vi "步进电机控制.vi"() -> ()   [LabVIEW 2015]
doc: "本范例使用Labview作为F4-Pro上位机控制步进电机.,可以使用速度模式,点动模式控制步进电机,同时检测限位开关的状态,可以配置通用输出端口的电平."
uses:
  <vilib>/Platform/browser.llb/Open URL in Default Browser (string).vi
  lib/pcomm/PCOMM.lvlib
panel:
  out "字符串 5":string="位置速度"
  out "字符串 4":string="运动控制"
  out "字符串 3":string="通用输入输出"
  out "字符串 2":string="运动模式"
  in  "刷新按钮":bool
  out "字符串":string="串口设置"
  in  "速度调节":sgl(knob) caption="速度旋钮" min=-600 max=600 scale=-600.0..600.0 scale format="%#_3f"
  in  "打开/关闭串口":bool
  in  "串口号":i32(ring)=1 items=["COM1 通信端口 (COM1)"=1, "COM2 ELTIMA Virtual Serial Port (COM2->COM3)"=2, "COM3 ELTIMA Virtual Serial Port (COM3->COM2)"=3, "COM8 USB-SERIAL CH340 (COM8)"=8]
  in  "波特率":i32(ring)=16 items=["1800"=8, "2400"=9, "4800"=10, "7200"=11, "9600"=12, "19200"=13, "38400"=14, "57600"=15, "115200"=16, "230400"=17, "460800"=18, "921600"=19]
  in  "数据比特":i32(ring)=3 caption="数据位" items=["5", "6", "7", "8"]
  in  "停止位":i32(ring) items=["1"=0, "2"=4]
  in  "奇偶校验":i32(ring) caption="校   验" items=["None"=0, "Odd"=8, "Even"=24, "Mark"=40, "Space"=56]
  in  "发送位置":bool
  in  "细分数":u32(ring)=32 items=["1"=1, "2"=2, "4"=4, "8"=8, "16"=16, "32"=32, "64"=64, "128"=128]
  out "圈数":sgl
  in  "脉冲数":u32 step=1
  in  "Out4":T1
  in  "Out3":T1
  in  "Out2":T1
  in  "Out1":T1
  out "IN3":bool caption="正极限"
  out "IN1":bool caption="原点检测"
  out "IN2":bool caption="负极限"
  in  "响应测试":bool
  in  "停止按钮":bool
  in  "点动控制":bool
  in  "接收:":string="硬石电子http://www.ing10bbs.com/\n            携手合作,共创未来\n"
  in  "速度位置选择":enum32{"未选择", "速度模式", "位置模式"}(radio)
  # "概述：Labview控制步进电机例程\n要求：PC已安装串口驱动，F4-Pro已下载配套例程.\n操作步骤：\n1.  使用USB线连接到F4-Pro的调试串口接口。\n2.  确保串口号为连接到F4-Pro的串口。\n3.  配置波特率等信息，F4-Pro通信配置是115200-8-None-1。\n4.  打开串口。\n5.  点击响应测试测试连接，文本框提示连接成功。"
  # "6.  选择速度模式或者位置模式\n7.  如果选择速度模式,则拖动速度旋钮，设置速度，\n    也可以直接输入速度值。\n8.  如果选择位置模式,则设置脉冲数和细分数，点击发送位置按钮。\n9.  按下点动控制按钮，则电机转动，松开按钮则停止，\n     速度值为旋钮所设置的速度值。\n10. 点击Out1~4，可以控制通用输出端口电平\n11. IN1~3指示通用输入1~3的电平状态"
  # "RPM"
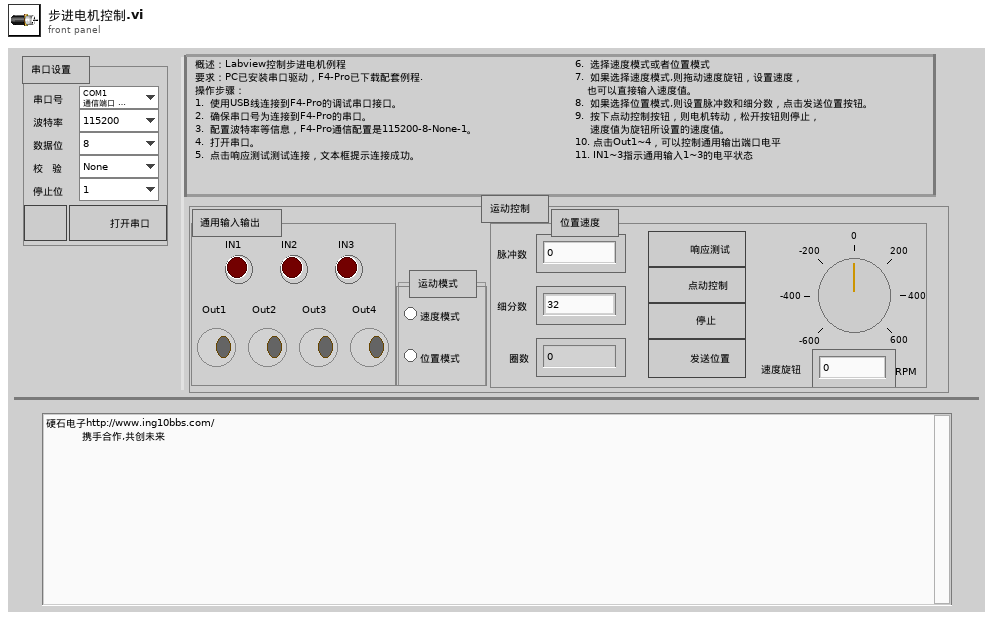
[diagram p1: front panel]
types:
  T1 = typedef "控件_通用输出.ctl" = bool
  T2 = enum8{"Enabled", "Disabled", "Disabled and Grayed Out"}
  T3 = typedef "控件 1" = bool
  T4 = typedef "LVRectTypeDef.ctl" = cluster{"Left":i16, "Top":i16, "Right":i16, "Bottom":i16}
  T5 = typedef "LVPointTypeDef.ctl" = cluster{"Horizontal":i16, "Vertical":i16}
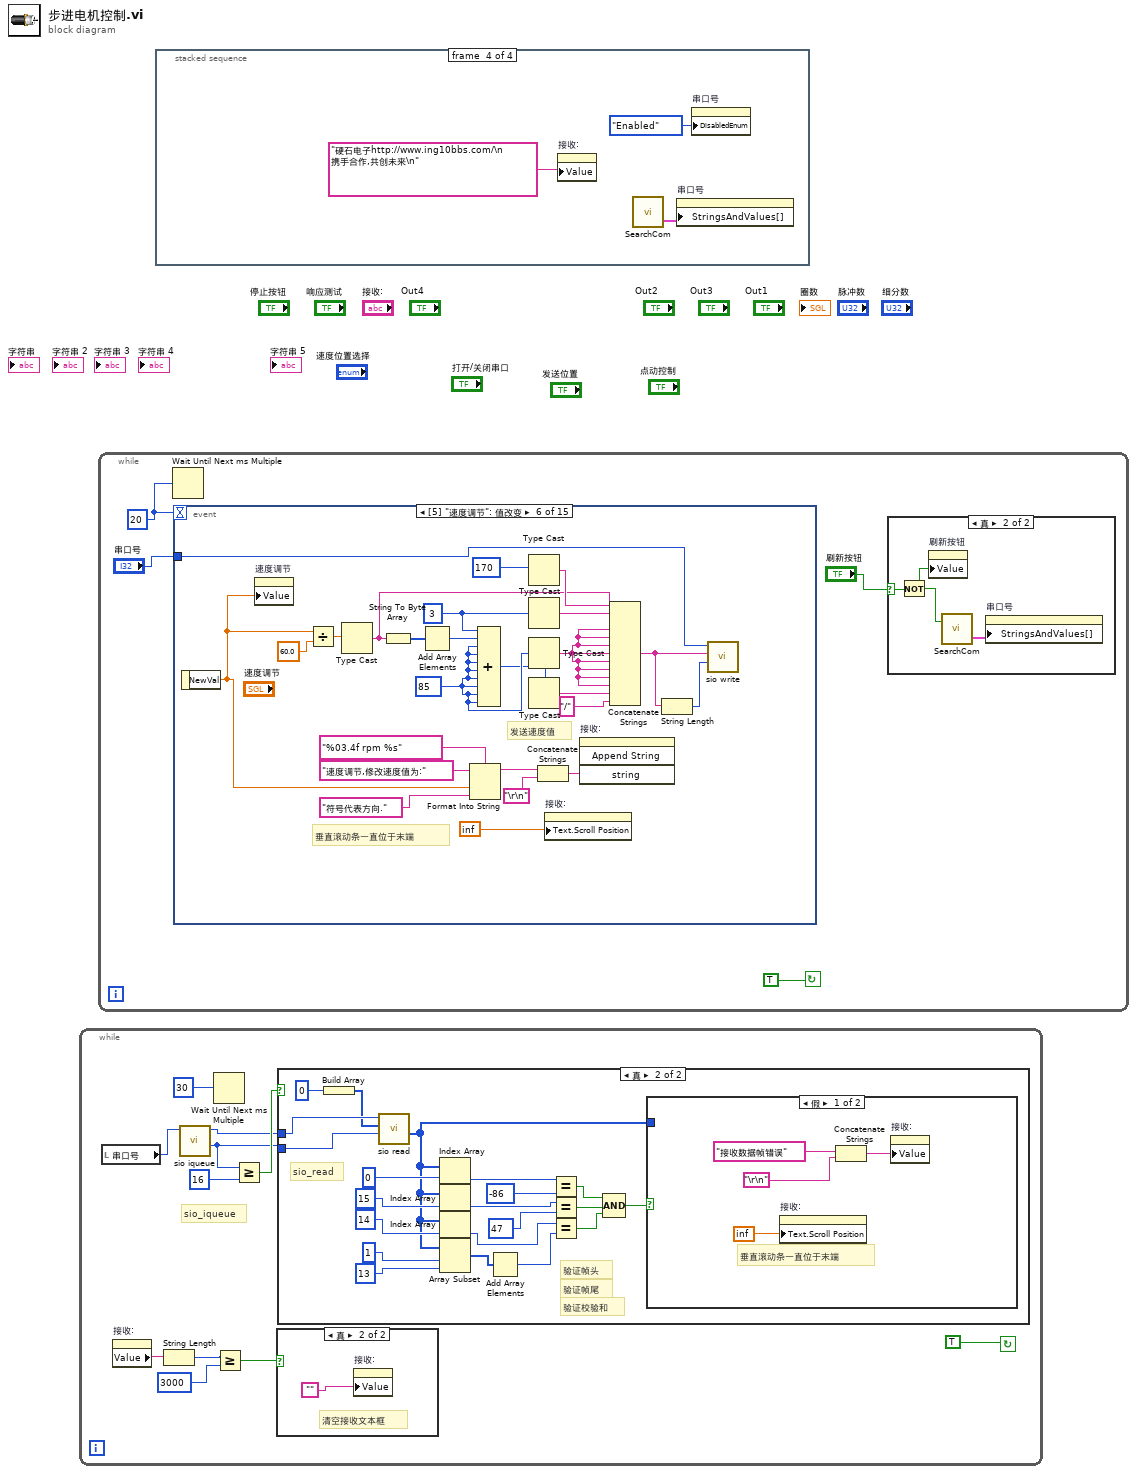
[diagram p0: block diagram]
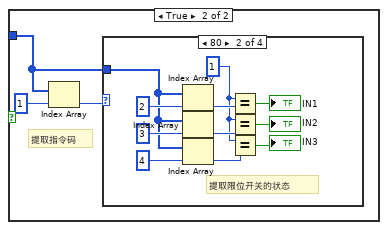
[diagram p4: hidden frame]
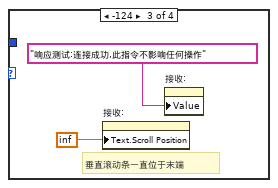
[diagram p6: hidden frame]
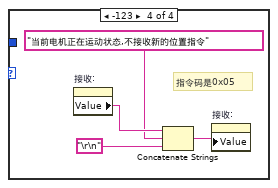
[diagram p7: hidden frame]
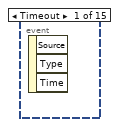
[diagram p9: hidden frame]
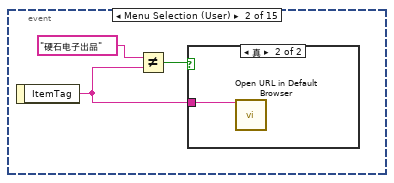
[diagram p10: hidden frame]
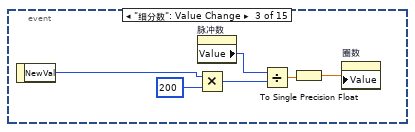
[diagram p12: hidden frame]
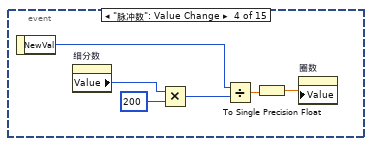
[diagram p13: hidden frame]
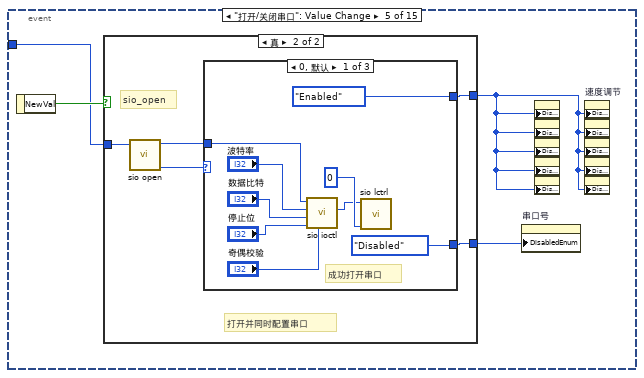
[diagram p14: hidden frame]
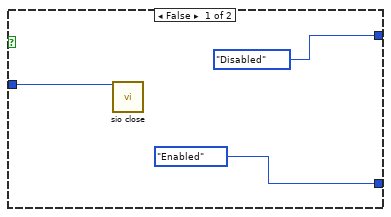
[diagram p15: hidden frame]
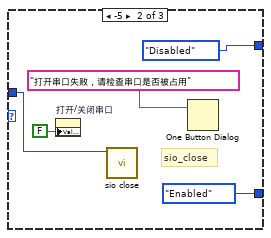
[diagram p16: hidden frame]
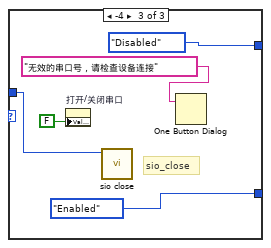
[diagram p17: hidden frame]
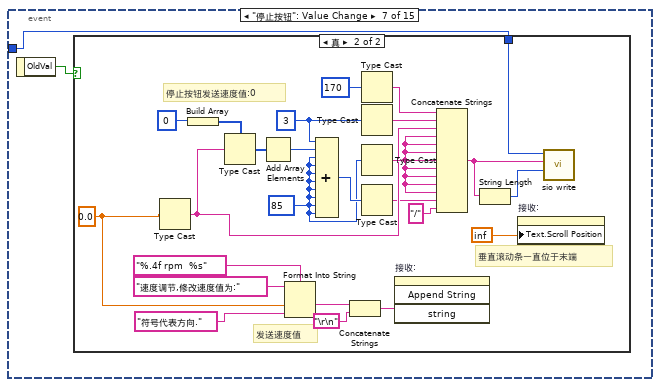
[diagram p18: hidden frame]
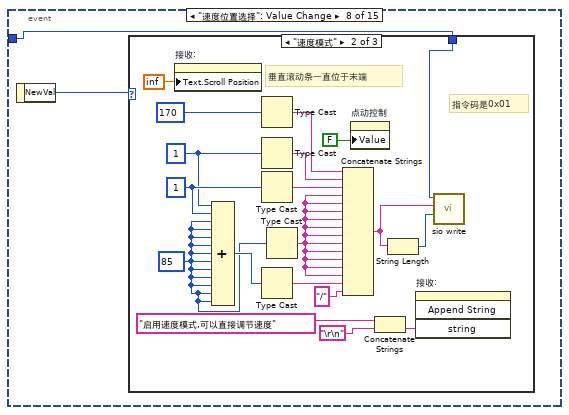
[diagram p20: hidden frame]
diagram:
  n1 = while {
    stop <- TRUE continue-if-true
    # "sio_iqueue"
    n2 = local read "串口号"() -> (w2:i32)
    n3 = property on="接收:" class="Str"() -> ("Value"=w3:string)  [unwired: 2 in, 2 out]
    n4 = String Length(string=w3) -> (length=w4:i32)
    n5 = call "sio iqueue.vi"("port"=w2) -> ("len"=w7:i32, "port"=w1:i32)  [unwired: 8 in, 1 out]
    n6 = Wait Until Next ms Multiple(millisecond multiple=u32 30) -> ()  [unwired: 1 out]
    n7 = Greater Or Equal?(x=w4, y=3000) -> (x >= y?=w5:bool)
    n8 = Greater Or Equal?(x=w7, y=16) -> (x >= y?=w8:bool)
    n9 = case shown="真" w5 {
      frame False {
      }
      frame True {
        # "清空接收文本框"
        n10 = property on="接收:" class="Str"("Value"="") -> ()  [unwired: 2 in, 2 out]
      }
    }
    n11 = case shown="真" w8 {
      tunnel: w1 -> [_ w15]
      tunnel: w7 -> [_ w13]
      frame False {
      }
      frame True {
        # "sio_read"
        # "验证帧尾"
        # "验证校验和"
        # "验证帧头"
        n12 = Build Array(i8 0) -> (w14:i8[])
        n13 = call "sio read.vi"("len"=w13, "buf"=w14, "port"=w15) -> ("buf out"=w16:i8[])  [unwired: 4 in, 3 out]
        n14 = Index Array(array=w16, index=0) -> (element=w31:i8)
        n15 = Index Array(array=w16, index=15) -> (element=w18:i8)
        n16 = Index Array(array=w16, index=14) -> (element=w20:i8)
        n17 = Array Subset(array=w16, index=1, length=13) -> (w24:i8[])
        n18 = Add Array Elements(numeric array=w24) -> (sum=w19:i8)
        n19 = Equal?(x=w31, y=i8 -86) -> (x = y?=w29:bool)
        n20 = Equal?(x=w18, y=i8 47) -> (x = y?=w26:bool)
        n21 = Equal?(x=w20, y=w19) -> (x = y?=w22:bool)
        n22 = Compound Arithmetic op=AND ("复合运算")(w29, w26, w22) -> (w33:bool)
        n23 = case shown="假" w33 {
          tunnel: w16 -> [_ w38]
          frame False {
            # "垂直滚动条一直位于末端"
            n24 = property on="接收:" class="Str"("Text.Scroll Position"=inf) -> ()  [unwired: 2 in, 2 out]
            n25 = Concatenate Strings("接收数据帧错误", "\r\n") -> (w35:string)
            n26 = property on="接收:" class="Str"("Value"=w35) -> ()  [unwired: 2 in, 2 out]
          }
          frame True {
            # "提取指令码"
            n27 = Index Array(array=w38, index=1) -> (element=w39:i8)
            n28 = case shown="80" w39 {
              tunnel: w38 -> [_ w44 _ _]
              frame Default {
                # "指令码0x00,无效"
              }
              frame -128 {
                w41 = i8 1
                # "提取限位开关的状态"
                n29 = Index Array(array=w44, index=2) -> (element=w47:i8)
                n30 = Index Array(array=w44, index=3) -> (element=w43:i8)
                n31 = Index Array(array=w44, index=4) -> (element=w42:i8)
                n32 = Equal?(x=w41, y=w47) -> (x = y?=→"IN1":bool)
                n33 = Equal?(x=w41, y=w43) -> (x = y?=→"IN2":bool)
                n34 = Equal?(x=w41, y=w42) -> (x = y?=→"IN3":bool)
              }
              frame -124 {
                # "垂直滚动条一直位于末端"
                n35 = property on="接收:" class="Str"("Text.Scroll Position"=inf) -> ()  [unwired: 2 in, 2 out]
                n36 = property on="接收:" class="Str"("Value"="响应测试:连接成功,此指令不影响任何操作") -> ()  [unwired: 2 in, 2 out]
              }
              frame -123 {
                # "指令码是0x05"
                n37 = property on="接收:" class="Str"() -> ("Value"=w57:string)  [unwired: 2 in, 2 out]
                n38 = Concatenate Strings(w57, "当前电机正在运动状态,不接收新的位置指令", "\r\n") -> (w56:string)
                n39 = property on="接收:" class="Str"("Value"=w56) -> ()  [unwired: 2 in, 2 out]
              }
            }
          }
        }
      }
    }
  }
  n40 = while {
    stop <- TRUE continue-if-true
    w60 = 20
    n41 = Wait Until Next ms Multiple(millisecond multiple=w60) -> ()  [unwired: 1 out]
    n42 = event shown="[5] \"速度调节\": 值改变" {
      selector: _ -> [_ _ _ _ _ _ _ _ _ _ _ _ _ _ _]
      dyn-events: _ -> [_ _ _ _ _ _ _ _ _ _ _ _ _ _ _]
      timeout: w60 -> [_ _ _ _ _ _ _ _ _ _ _ _ _ _ _]
      tunnel: "串口号" -> [_ _ _ _ w82 w114 w137 w164 w221 w261 w277 w305 w333 w361 w388]
      event Timeout {
        n43 = event-data() -> ()  [unwired: 1 in, 3 out]
      }
      event Menu Selection (User) {
        n44 = event-data() -> ("ItemTag"=w65:string)  [unwired: 1 in]
        n45 = Not Equal?(x="硬石电子出品", y=w65) -> (x != y?=w66:bool)
        n46 = case shown="真" w66 {
          tunnel: w65 -> [_ w68]
          frame False {
          }
          frame True {
            n47 = call-poly <vilib>:"Open URL in Default Browser.vi"("URL"=w68) -> ()  [unwired: 5 in, 2 out]
          }
        }
      }
      event "细分数": Value Change {
        n48 = event-data() -> ("NewVal"=w69:u32)  [unwired: 1 in]
        n49 = Multiply(x=w69, y=200) -> (x*y=w72:u32)
        n50 = property on="脉冲数" class="DigNum (严格)"() -> ("Value"=w74:u32)  [unwired: 2 in, 2 out]
        n51 = Divide(x=w74, y=w72) -> (x/y=w71:dbl)
        n52 = To Single Precision Float(number=w71) -> (single precision float=w70:sgl)
        n53 = property on="圈数" class="DigNum (严格)"("Value"=w70) -> ()  [unwired: 2 in, 2 out]
      }
      event "脉冲数": Value Change {
        n54 = event-data() -> ("NewVal"=w75:u32)  [unwired: 1 in]
        n55 = property on="细分数" class="Ring (严格)"() -> ("Value"=w80:u32)  [unwired: 2 in, 2 out]
        n56 = Multiply(x=w80, y=200) -> (x*y=w78:u32)
        n57 = Divide(x=w75, y=w78) -> (x/y=w77:dbl)
        n58 = To Single Precision Float(number=w77) -> (single precision float=w76:sgl)
        n59 = property on="圈数" class="DigNum (严格)"("Value"=w76) -> ()  [unwired: 2 in, 2 out]
      }
      event "打开/关闭串口": Value Change {
        n60 = event-data() -> ("NewVal"=w84:bool)  [unwired: 1 in]
        n61 = case shown="真" w84 {
          tunnel: [T2."Enabled" w92] -> w83
          tunnel: [T2."Disabled" w91] -> w81
          tunnel: w82 -> [w85 w90]
          frame False {
            n62 = call "sio close.vi"("port"=w85) -> ()  [unwired: 9 in, 2 out]
          }
          frame True {
            # "sio_open"
            # "打开并同时配置串口"
            n63 = call "sio open.vi"("port"=w90) -> ("port"=w88:i32, "Status"=w89:i32)  [unwired: 6 in]
            n64 = case shown="0, 默认" w89 {
              tunnel: w88 -> [w97 w102 w107]
              tunnel: [T2."Enabled" T2."Disabled" T2."Disabled"] -> w91
              tunnel: [T2."Disabled" T2."Enabled" T2."Enabled"] -> w92
              frame 0, Default {
                # "成功打开串口"
                n65 = call "sio ioctl.vi"("parity"="奇偶校验", "stop bits"="停止位", "data bits"="数据比特", "baud"="波特率", "port"=w97) -> ("port"=w93:i32)  [unwired: 5 in, 1 out]
                n66 = call "sio lctrl.vi"("mode"=0, "port"=w93) -> ()  [unwired: 8 in, 2 out]
              }
              frame -5 {
                # "sio_close"
                n67 = property on="打开/关闭串口" class="Bool (严格)"("Value"=FALSE) -> ()  [unwired: 2 in, 2 out]
                n68 = call "sio close.vi"("port"=w102) -> ()  [unwired: 9 in, 2 out]
                n69 = One Button Dialog(message="打开串口失败，请检查串口是否被占用") -> ()  [unwired: 1 in, 1 out]
              }
              frame -4 {
                # "sio_close"
                n70 = property on="打开/关闭串口" class="Bool (严格)"("Value"=FALSE) -> ()  [unwired: 2 in, 2 out]
                n71 = call "sio close.vi"("port"=w107) -> ()  [unwired: 9 in, 2 out]
                n72 = One Button Dialog(message="无效的串口号，请检查设备连接") -> ()  [unwired: 1 in, 1 out]
              }
            }
          }
        }
        n73 = property on="串口号" class="Ring (严格)"("DisabledEnum"=w83) -> ()  [unwired: 2 in, 2 out]
        n74 = property on="点动控制" class="Bool (严格)"("DisabledEnum"=w81) -> ()  [unwired: 2 in, 2 out]
        n75 = property on="Output2" class="Bool (严格)"("DisabledEnum"=w81) -> ()  [unwired: 2 in, 2 out]
        n76 = property on="速度位置选择" class="RadioBtnsControl (严格)"("DisabledEnum"=w81) -> ()  [unwired: 2 in, 2 out]
        n77 = property on="停止按钮" class="Bool (严格)"("DisabledEnum"=w81) -> ()  [unwired: 2 in, 2 out]
        n78 = property on="Output4" class="Bool (严格)"("DisabledEnum"=w81) -> ()  [unwired: 2 in, 2 out]
        n79 = property on="速度调节" class="Knob (严格)"("DisabledEnum"=w81) -> ()  [unwired: 2 in, 2 out]
        n80 = property on="Output3" class="Bool (严格)"("DisabledEnum"=w81) -> ()  [unwired: 2 in, 2 out]
        n81 = property on="发送位置" class="Bool (严格)"("DisabledEnum"=w81) -> ()  [unwired: 2 in, 2 out]
        n82 = property on="响应测试" class="Bool (严格)"("DisabledEnum"=w81) -> ()  [unwired: 2 in, 2 out]
        n83 = property on="Output1" class="Bool (严格)"("DisabledEnum"=w81) -> ()  [unwired: 2 in, 2 out]
      }
      event "速度调节": Value Change {
        w124 = u8 85
        w123 = u8 3
        # "垂直滚动条一直位于末端"
        # "发送速度值"
        n84 = event-data() -> ("NewVal"=w117:sgl)  [unwired: 1 in]
        n85 = property on="速度调节" class="Knob (严格)"("Value"=w117) -> ()  [unwired: 2 in, 2 out]
        n86 = Divide(x=w117, y=sgl 60.0) -> (x/y=w136:sgl)
        n87 = Type Cast(x=w136) -> (*(type *) &x=w113:string)  [unwired: 1 in]
        n88 = String To Byte Array(string=w113) -> (unsigned byte array=w112:u8[])
        n89 = Add Array Elements(numeric array=w112) -> (sum=w128:u8)
        n90 = Format Into String(format string="%03.4f rpm %s", initial string="速度调节,修改速度值为:", w117, "符号代表方向.") -> (resulting string=w132:string)  [unwired: 1 in, 1 out]
        n91 = Compound Arithmetic op=ADD(w123, w128, w124, w124, w124, w124, w124, w124, w124, w124) -> (w120:u8)
        n92 = Type Cast(x=u8 170) -> (*(type *) &x=w121:string)  [unwired: 1 in]
        n93 = Type Cast(x=w123) -> (*(type *) &x=w122:string)  [unwired: 1 in]
        n94 = Type Cast(x=w124) -> (*(type *) &x=w126:string)  [unwired: 1 in]
        n95 = Type Cast(x=w120) -> (*(type *) &x=w127:string)  [unwired: 1 in]
        n96 = Concatenate Strings(w132, "\r\n") -> (w118:string)
        n97 = property on="接收:" class="Str"("Text.Scroll Position"=inf) -> ()  [unwired: 2 in, 2 out]
        n98 = invoke on="接收:" class="Str" method="Append String"("string"=w118) -> ()  [unwired: 3 in, 4 out]
        n99 = Concatenate Strings(w121, w122, w113, w126, w126, w126, w126, w126, w126, w126, w126, w127, "/") -> (w116:string)
        n100 = String Length(string=w116) -> (length=w115:i32)
        n101 = call "sio write.vi"("len"=w115, "buf"=w116, "port"=w114) -> ()  [unwired: 6 in, 3 out]
      }
      event "停止按钮": Value Change {
        n102 = event-data() -> ("OldVal"=w138:bool)  [unwired: 1 in]
        n103 = case shown="真" w138 {
          tunnel: w137 -> [_ w141]
          frame False {
          }
          frame True {
            w158 = u8 85
            w159 = u8 3
            w142 = sgl 0.0
            # "垂直滚动条一直位于末端"
            # "发送速度值"
            # "停止按钮发送速度值:0"
            n104 = Type Cast(x=w142) -> (*(type *) &x=w151:string)  [unwired: 1 in]
            n105 = Build Array(u8 0) -> (w154:u8[])
            n106 = Type Cast(type=w154, x=w151) -> (*(type *) &x=w153:u8[])
            n107 = Add Array Elements(numeric array=w153) -> (sum=w152:u8)
            n108 = Format Into String(format string="%.4f rpm  %s", initial string="速度调节,修改速度值为:", w142, "符号代表方向.") -> (resulting string=w145:string)  [unwired: 1 in, 1 out]
            n109 = Compound Arithmetic op=ADD(w159, w152, w158, w158, w158, w158, w158, w158, w158, w158) -> (w162:u8)
            n110 = Concatenate Strings(w145, "\r\n") -> (w143:string)
            n111 = Type Cast(x=u8 170) -> (*(type *) &x=w161:string)  [unwired: 1 in]
            n112 = Type Cast(x=w159) -> (*(type *) &x=w160:string)  [unwired: 1 in]
            n113 = Type Cast(x=w158) -> (*(type *) &x=w156:string)  [unwired: 1 in]
            n114 = Type Cast(x=w162) -> (*(type *) &x=w150:string)  [unwired: 1 in]
            n115 = invoke on="接收:" class="Str" method="Append String"("string"=w143) -> ()  [unwired: 3 in, 4 out]
            n116 = Concatenate Strings(w161, w160, w151, w156, w156, w156, w156, w156, w156, w156, w156, w150, "/") -> (w140:string)
            n117 = String Length(string=w140) -> (length=w139:i32)
            n118 = property on="接收:" class="Str"("Text.Scroll Position"=inf) -> ()  [unwired: 2 in, 2 out]
            n119 = call "sio write.vi"("len"=w139, "buf"=w140, "port"=w141) -> ()  [unwired: 6 in, 3 out]
          }
        }
      }
      event "速度位置选择": Value Change {
        n120 = event-data() -> ("NewVal"=w165:enum32{"未选择", "速度模式", "位置模式"})  [unwired: 1 in]
        n121 = case shown="\"速度模式\"" w165 {
          tunnel: w164 -> [w168 w186 w205]
          frame "未选择", Default {
            w169 = u8 85
            w174 = u8 0
            w175 = u8 1
            # "垂直滚动条一直位于末端"
            # "速度模式,指令码0x01"
            n122 = Compound Arithmetic op=ADD(w175, w174, w169, w169, w169, w169, w169, w169, w169, w169, w169, w169, w169) -> (w181:u8)
            n123 = Concatenate Strings("停止速度位置模式", "\r\n") -> (w170:string)
            n124 = Type Cast(x=u8 170) -> (*(type *) &x=w180:string)  [unwired: 1 in]
            n125 = Type Cast(x=w175) -> (*(type *) &x=w179:string)  [unwired: 1 in]
            n126 = Type Cast(x=w174) -> (*(type *) &x=w178:string)  [unwired: 1 in]
            n127 = Type Cast(x=w169) -> (*(type *) &x=w183:string)  [unwired: 1 in]
            n128 = Type Cast(x=w181) -> (*(type *) &x=w177:string)  [unwired: 1 in]
            n129 = invoke on="接收:" class="Str" method="Append String"("string"=w170) -> ()  [unwired: 3 in, 4 out]
            n130 = Concatenate Strings(w180, w179, w178, w183, w183, w183, w183, w183, w183, w183, w183, w183, w183, w183, w177, "/") -> (w167:string)
            n131 = String Length(string=w167) -> (length=w166:i32)
            n132 = property on="接收:" class="Str"("Text.Scroll Position"=inf) -> ()  [unwired: 2 in, 2 out]
            n133 = call "sio write.vi"("len"=w166, "buf"=w167, "port"=w168) -> ()  [unwired: 6 in, 3 out]
          }
          frame "速度模式" {
            w191 = u8 85
            w199 = u8 1
            w193 = u8 1
            # "垂直滚动条一直位于末端"
            # "指令码是0x01"
            n134 = property on="接收:" class="Str"("Text.Scroll Position"=inf) -> ()  [unwired: 2 in, 2 out]
            n135 = Compound Arithmetic op=ADD(w193, w199, w191, w191, w191, w191, w191, w191, w191, w191, w191, w191, w191) -> (w200:u8)
            n136 = Type Cast(x=u8 170) -> (*(type *) &x=w202:string)  [unwired: 1 in]
            n137 = Type Cast(x=w193) -> (*(type *) &x=w201:string)  [unwired: 1 in]
            n138 = Type Cast(x=w199) -> (*(type *) &x=w198:string)  [unwired: 1 in]
            n139 = Type Cast(x=w200) -> (*(type *) &x=w196:string)  [unwired: 1 in]
            n140 = Type Cast(x=w191) -> (*(type *) &x=w197:string)  [unwired: 1 in]
            n141 = Concatenate Strings(w202, w201, w198, w197, w197, w197, w197, w197, w197, w197, w197, w197, w197, w197, w196, "/") -> (w185:string)
            n142 = property on="点动控制" class="Bool (严格)"("Value"=FALSE) -> ()  [unwired: 2 in, 2 out]
            n143 = Concatenate Strings("启用速度模式,可以直接调节速度", "\r\n") -> (w187:string)
            n144 = String Length(string=w185) -> (length=w184:i32)
            n145 = invoke on="接收:" class="Str" method="Append String"("string"=w187) -> ()  [unwired: 3 in, 4 out]
            n146 = call "sio write.vi"("len"=w184, "buf"=w185, "port"=w186) -> ()  [unwired: 6 in, 3 out]
          }
          frame "位置模式" {
            w207 = u8 85
            w217 = u8 2
            w211 = u8 1
            # "垂直滚动条一直位于末端"
            # "指令码是0x01"
            n147 = property on="接收:" class="Str"("Text.Scroll Position"=inf) -> ()  [unwired: 2 in, 2 out]
            n148 = Compound Arithmetic op=ADD(w211, w217, w207, w207, w207, w207, w207, w207, w207, w207, w207, w207, w207) -> (w218:u8)
            n149 = Type Cast(x=u8 170) -> (*(type *) &x=w220:string)  [unwired: 1 in]
            n150 = Type Cast(x=w211) -> (*(type *) &x=w219:string)  [unwired: 1 in]
            n151 = Type Cast(x=w217) -> (*(type *) &x=w216:string)  [unwired: 1 in]
            n152 = Type Cast(x=w207) -> (*(type *) &x=w215:string)  [unwired: 1 in]
            n153 = Type Cast(x=w218) -> (*(type *) &x=w214:string)  [unwired: 1 in]
            n154 = Concatenate Strings(w220, w219, w216, w215, w215, w215, w215, w215, w215, w215, w215, w215, w215, w215, w214, "/") -> (w204:string)
            n155 = String Length(string=w204) -> (length=w203:i32)
            n156 = call "sio write.vi"("len"=w203, "buf"=w204, "port"=w205) -> ()  [unwired: 6 in, 3 out]
            n157 = Concatenate Strings("启用位置模式,确定速度,脉冲数和细分数后点击发送位置", "\r\n") -> (w206:string)
            n158 = invoke on="接收:" class="Str" method="Append String"("string"=w206) -> ()  [unwired: 3 in, 4 out]
          }
        }
      }
      event "点动控制": Value Change {
        n159 = event-data() -> ("NewVal"=w222:bool)  [unwired: 1 in, 5 out]
        n160 = case shown="假" w222 {
          tunnel: w221 -> [w226 w245]
          frame False {
            w232 = u8 85
            w233 = u8 0
            w234 = u8 2
            # "垂直滚动条一直位于末端"
            # "指令码是0x02"
            n161 = property on="接收:" class="Str"("Text.Scroll Position"=inf) -> ()  [unwired: 2 in, 2 out]
            n162 = Compound Arithmetic op=ADD(w234, w233, w232, w232, w232, w232, w232, w232, w232, w232, w232, w232, w232) -> (w240:u8)
            n163 = Type Cast(x=u8 170) -> (*(type *) &x=w239:string)  [unwired: 1 in]
            n164 = property on="接收:" class="Str"() -> ("Value"=w231:string)  [unwired: 2 in, 2 out]
            n165 = Type Cast(x=w234) -> (*(type *) &x=w238:string)  [unwired: 1 in]
            n166 = Type Cast(x=w233) -> (*(type *) &x=w237:string)  [unwired: 1 in]
            n167 = Type Cast(x=w232) -> (*(type *) &x=w242:string)  [unwired: 1 in]
            n168 = Type Cast(x=w240) -> (*(type *) &x=w236:string)  [unwired: 1 in]
            n169 = Concatenate Strings(w231, "点动控制,已停止 ", "\r\n") -> (w230:string)
            n170 = Concatenate Strings(w239, w238, w237, w242, w242, w242, w242, w242, w242, w242, w242, w242, w242, w242, w236, "/") -> (w225:string)
            n171 = property on="接收:" class="Str"("Value"=w230) -> ()  [unwired: 2 in, 2 out]
            n172 = String Length(string=w225) -> (length=w224:i32)
            n173 = call "sio write.vi"("len"=w224, "buf"=w225, "port"=w226) -> ()  [unwired: 6 in, 3 out]
          }
          frame True {
            w250 = u8 85
            w251 = u8 1
            w252 = u8 2
            # "垂直滚动条一直位于末端"
            # "点动模式控制"
            n174 = Compound Arithmetic op=ADD(w252, w251, w250, w250, w250, w250, w250, w250, w250, w250, w250, w250, w250) -> (w258:u8)
            n175 = Concatenate Strings("点动控制,释放按钮即停止", "\r\n") -> (w246:string)
            n176 = Type Cast(x=w252) -> (*(type *) &x=w256:string)  [unwired: 1 in]
            n177 = Type Cast(x=w251) -> (*(type *) &x=w255:string)  [unwired: 1 in]
            n178 = Type Cast(x=w250) -> (*(type *) &x=w260:string)  [unwired: 1 in]
            n179 = Type Cast(x=w258) -> (*(type *) &x=w254:string)  [unwired: 1 in]
            n180 = Type Cast(x=u8 170) -> (*(type *) &x=w257:string)  [unwired: 1 in]
            n181 = invoke on="接收:" class="Str" method="Append String"("string"=w246) -> ()  [unwired: 3 in, 4 out]
            n182 = Concatenate Strings(w257, w256, w255, w260, w260, w260, w260, w260, w260, w260, w260, w260, w260, w260, w254, "/") -> (w243:string)
            n183 = String Length(string=w243) -> (length=w244:i32)
            n184 = property on="接收:" class="Str"("Text.Scroll Position"=inf) -> ()  [unwired: 2 in, 2 out]
            n185 = call "sio write.vi"("len"=w244, "buf"=w243, "port"=w245) -> ()  [unwired: 6 in, 3 out]
          }
        }
        n186 = property on="速度位置选择" class="RadioBtnsControl (严格)"("Value"=enum32{"未选择", "速度模式", "位置模式"}."未选择") -> ()  [unwired: 2 in, 2 out]
      }
      event "响应测试": Value Change {
        n187 = event-data() -> ("OldVal"=w262:bool)  [unwired: 1 in]
        n188 = case shown="真" w262 {
          tunnel: w261 -> [_ w265]
          frame False {
          }
          frame True {
            w267 = u8 85
            w268 = u8 4
            # "响应测试"
            n189 = Compound Arithmetic op=ADD(w268, w267, w267, w267, w267, w267, w267, w267, w267, w267, w267, w267, w267) -> (w272:u8)
            n190 = Type Cast(x=u8 170) -> (*(type *) &x=w274:string)  [unwired: 1 in]
            n191 = Type Cast(x=w268) -> (*(type *) &x=w273:string)  [unwired: 1 in]
            n192 = Type Cast(x=w267) -> (*(type *) &x=w266:string)  [unwired: 1 in]
            n193 = Type Cast(x=w272) -> (*(type *) &x=w271:string)  [unwired: 1 in]
            n194 = Concatenate Strings(w274, w273, w266, w266, w266, w266, w266, w266, w266, w266, w266, w266, w266, w266, w271, "/") -> (w264:string)
            n195 = String Length(string=w264) -> (length=w263:i32)
            n196 = call "sio write.vi"("len"=w263, "buf"=w264, "port"=w265) -> ()  [unwired: 6 in, 3 out]
          }
        }
      }
      event Value Change {
        w295 = u8 85
        w296 = u8 6
        n197 = event-data() -> ("NewVal"=w279:T1)  [unwired: 1 in]
        n198 = property on="Output2" class="Bool (严格)"() -> ("Value"=w282:T3)  [unwired: 2 in, 2 out]
        n199 = property on="Output4" class="Bool (严格)"() -> ("Value"=w280:T3)  [unwired: 2 in, 2 out]
        n200 = property on="Output3" class="Bool (严格)"() -> ("Value"=w281:T3)  [unwired: 2 in, 2 out]
        n201 = Boolean To (0,1)(Boolean=w279) -> (0, 1=w290:i16)
        n202 = Boolean To (0,1)(Boolean=w282) -> (0, 1=w288:i16)
        n203 = Boolean To (0,1)(Boolean=w281) -> (0, 1=w286:i16)
        n204 = Boolean To (0,1)(Boolean=w280) -> (0, 1=w284:i16)
        n205 = To Unsigned Byte Integer(number=w290) -> (unsigned 8bit integer=w289:u8)
        n206 = To Unsigned Byte Integer(number=w288) -> (unsigned 8bit integer=w287:u8)
        n207 = To Unsigned Byte Integer(number=w286) -> (unsigned 8bit integer=w285:u8)
        n208 = To Unsigned Byte Integer(number=w284) -> (unsigned 8bit integer=w283:u8)
        n209 = Compound Arithmetic op=ADD(w296, w289, w287, w285, w283, w295, w295, w295, w295, w295, w295, w295, w295) -> (w300:u8)
        n210 = Type Cast(x=u8 170) -> (*(type *) &x=w302:string)  [unwired: 1 in]
        n211 = Type Cast(x=w296) -> (*(type *) &x=w301:string)  [unwired: 1 in]
        n212 = Type Cast(x=w289) -> (*(type *) &x=w293:string)  [unwired: 1 in]
        n213 = Type Cast(x=w287) -> (*(type *) &x=w292:string)  [unwired: 1 in]
        n214 = Type Cast(x=w285) -> (*(type *) &x=w291:string)  [unwired: 1 in]
        n215 = Type Cast(x=w283) -> (*(type *) &x=w278:string)  [unwired: 1 in]
        n216 = Type Cast(x=w295) -> (*(type *) &x=w294:string)  [unwired: 1 in]
        n217 = Type Cast(x=w300) -> (*(type *) &x=w299:string)  [unwired: 1 in]
        n218 = Concatenate Strings(w302, w301, w293, w292, w291, w278, w294, w294, w294, w294, w294, w294, w294, w294, w299, "/") -> (w276:string)
        n219 = String Length(string=w276) -> (length=w275:i32)
        n220 = call "sio write.vi"("len"=w275, "buf"=w276, "port"=w277) -> ()  [unwired: 6 in, 3 out]
      }
      event Value Change {
        w323 = u8 85
        w324 = u8 6
        n221 = event-data() -> ("NewVal"=w307:T1)  [unwired: 1 in]
        n222 = property on="Output1" class="Bool (严格)"() -> ("Value"=w306:T1)  [unwired: 2 in, 2 out]
        n223 = property on="Output3" class="Bool (严格)"() -> ("Value"=w310:T3)  [unwired: 2 in, 2 out]
        n224 = property on="Output4" class="Bool (严格)"() -> ("Value"=w309:T3)  [unwired: 2 in, 2 out]
        n225 = Boolean To (0,1)(Boolean=w306) -> (0, 1=w318:i16)
        n226 = Boolean To (0,1)(Boolean=w307) -> (0, 1=w316:i16)
        n227 = Boolean To (0,1)(Boolean=w310) -> (0, 1=w314:i16)
        n228 = Boolean To (0,1)(Boolean=w309) -> (0, 1=w312:i16)
        n229 = To Unsigned Byte Integer(number=w318) -> (unsigned 8bit integer=w317:u8)
        n230 = To Unsigned Byte Integer(number=w316) -> (unsigned 8bit integer=w315:u8)
        n231 = To Unsigned Byte Integer(number=w314) -> (unsigned 8bit integer=w313:u8)
        n232 = To Unsigned Byte Integer(number=w312) -> (unsigned 8bit integer=w311:u8)
        n233 = Compound Arithmetic op=ADD(w324, w317, w315, w313, w311, w323, w323, w323, w323, w323, w323, w323, w323) -> (w328:u8)
        n234 = Type Cast(x=u8 170) -> (*(type *) &x=w330:string)  [unwired: 1 in]
        n235 = Type Cast(x=w324) -> (*(type *) &x=w329:string)  [unwired: 1 in]
        n236 = Type Cast(x=w317) -> (*(type *) &x=w321:string)  [unwired: 1 in]
        n237 = Type Cast(x=w315) -> (*(type *) &x=w320:string)  [unwired: 1 in]
        n238 = Type Cast(x=w313) -> (*(type *) &x=w319:string)  [unwired: 1 in]
        n239 = Type Cast(x=w311) -> (*(type *) &x=w308:string)  [unwired: 1 in]
        n240 = Type Cast(x=w323) -> (*(type *) &x=w322:string)  [unwired: 1 in]
        n241 = Type Cast(x=w328) -> (*(type *) &x=w327:string)  [unwired: 1 in]
        n242 = Concatenate Strings(w330, w329, w321, w320, w319, w308, w322, w322, w322, w322, w322, w322, w322, w322, w327, "/") -> (w304:string)
        n243 = String Length(string=w304) -> (length=w303:i32)
        n244 = call "sio write.vi"("len"=w303, "buf"=w304, "port"=w305) -> ()  [unwired: 6 in, 3 out]
      }
      event Value Change {
        w351 = u8 85
        w352 = u8 6
        n245 = event-data() -> ("NewVal"=w335:T1)  [unwired: 1 in]
        n246 = property on="Output1" class="Bool (严格)"() -> ("Value"=w336:T1)  [unwired: 2 in, 2 out]
        n247 = property on="Output2" class="Bool (严格)"() -> ("Value"=w334:T1)  [unwired: 2 in, 2 out]
        n248 = property on="Output4" class="Bool (严格)"() -> ("Value"=w338:T3)  [unwired: 2 in, 2 out]
        n249 = Boolean To (0,1)(Boolean=w336) -> (0, 1=w346:i16)
        n250 = Boolean To (0,1)(Boolean=w334) -> (0, 1=w344:i16)
        n251 = Boolean To (0,1)(Boolean=w335) -> (0, 1=w342:i16)
        n252 = Boolean To (0,1)(Boolean=w338) -> (0, 1=w340:i16)
        n253 = To Unsigned Byte Integer(number=w346) -> (unsigned 8bit integer=w345:u8)
        n254 = To Unsigned Byte Integer(number=w344) -> (unsigned 8bit integer=w343:u8)
        n255 = To Unsigned Byte Integer(number=w342) -> (unsigned 8bit integer=w341:u8)
        n256 = To Unsigned Byte Integer(number=w340) -> (unsigned 8bit integer=w339:u8)
        n257 = Compound Arithmetic op=ADD(w352, w345, w343, w341, w339, w351, w351, w351, w351, w351, w351, w351, w351) -> (w356:u8)
        n258 = Type Cast(x=u8 170) -> (*(type *) &x=w358:string)  [unwired: 1 in]
        n259 = Type Cast(x=w352) -> (*(type *) &x=w357:string)  [unwired: 1 in]
        n260 = Type Cast(x=w345) -> (*(type *) &x=w349:string)  [unwired: 1 in]
        n261 = Type Cast(x=w343) -> (*(type *) &x=w348:string)  [unwired: 1 in]
        n262 = Type Cast(x=w341) -> (*(type *) &x=w347:string)  [unwired: 1 in]
        n263 = Type Cast(x=w339) -> (*(type *) &x=w337:string)  [unwired: 1 in]
        n264 = Type Cast(x=w351) -> (*(type *) &x=w350:string)  [unwired: 1 in]
        n265 = Type Cast(x=w356) -> (*(type *) &x=w355:string)  [unwired: 1 in]
        n266 = Concatenate Strings(w358, w357, w349, w348, w347, w337, w350, w350, w350, w350, w350, w350, w350, w350, w355, "/") -> (w332:string)
        n267 = String Length(string=w332) -> (length=w331:i32)
        n268 = call "sio write.vi"("len"=w331, "buf"=w332, "port"=w333) -> ()  [unwired: 6 in, 3 out]
      }
      event Value Change {
        w379 = u8 85
        w380 = u8 6
        n269 = event-data() -> ("NewVal"=w362:T1)  [unwired: 1 in]
        n270 = property on="Output1" class="Bool (严格)"() -> ("Value"=w365:T1)  [unwired: 2 in, 2 out]
        n271 = property on="Output2" class="Bool (严格)"() -> ("Value"=w364:T1)  [unwired: 2 in, 2 out]
        n272 = property on="Output3" class="Bool (严格)"() -> ("Value"=w363:T1)  [unwired: 2 in, 2 out]
        n273 = Boolean To (0,1)(Boolean=w365) -> (0, 1=w374:i16)
        n274 = Boolean To (0,1)(Boolean=w364) -> (0, 1=w372:i16)
        n275 = Boolean To (0,1)(Boolean=w363) -> (0, 1=w370:i16)
        n276 = Boolean To (0,1)(Boolean=w362) -> (0, 1=w368:i16)
        n277 = To Unsigned Byte Integer(number=w374) -> (unsigned 8bit integer=w373:u8)
        n278 = To Unsigned Byte Integer(number=w372) -> (unsigned 8bit integer=w371:u8)
        n279 = To Unsigned Byte Integer(number=w370) -> (unsigned 8bit integer=w369:u8)
        n280 = To Unsigned Byte Integer(number=w368) -> (unsigned 8bit integer=w367:u8)
        n281 = Compound Arithmetic op=ADD(w380, w373, w371, w369, w367, w379, w379, w379, w379, w379, w379, w379, w379) -> (w384:u8)
        n282 = Type Cast(x=u8 170) -> (*(type *) &x=w386:string)  [unwired: 1 in]
        n283 = Type Cast(x=w380) -> (*(type *) &x=w385:string)  [unwired: 1 in]
        n284 = Type Cast(x=w373) -> (*(type *) &x=w377:string)  [unwired: 1 in]
        n285 = Type Cast(x=w371) -> (*(type *) &x=w376:string)  [unwired: 1 in]
        n286 = Type Cast(x=w369) -> (*(type *) &x=w375:string)  [unwired: 1 in]
        n287 = Type Cast(x=w367) -> (*(type *) &x=w366:string)  [unwired: 1 in]
        n288 = Type Cast(x=w379) -> (*(type *) &x=w378:string)  [unwired: 1 in]
        n289 = Type Cast(x=w384) -> (*(type *) &x=w383:string)  [unwired: 1 in]
        n290 = Concatenate Strings(w386, w385, w377, w376, w375, w366, w378, w378, w378, w378, w378, w378, w378, w378, w383, "/") -> (w360:string)
        n291 = String Length(string=w360) -> (length=w359:i32)
        n292 = call "sio write.vi"("len"=w359, "buf"=w360, "port"=w361) -> ()  [unwired: 6 in, 3 out]
      }
      event "发送位置": Value Change {
        n293 = event-data() -> ("OldVal"=w387:bool)  [unwired: 1 in]
        n294 = case shown="真" w387 {
          tunnel: w388 -> [_ w391]
          frame False {
          }
          frame True {
            w406 = u8 85
            w407 = u8 5
            # "发送位置"
            n295 = property on="脉冲数" class="DigNum (严格)"() -> ("Value"=w396:u32)  [unwired: 2 in, 2 out]
            n296 = Number To Decimal String(number=w396) -> (decimal integer string=w395:string)  [unwired: 1 in]
            n297 = Build Array(u8 0) -> (w402:u8[])
            n298 = Type Cast(type=w402, x=w396) -> (*(type *) &x=w398:u8[])
            n299 = property on="接收:" class="Str"("Text.Scroll Position"=inf) -> ()  [unwired: 2 in, 2 out]
            n300 = Add Array Elements(numeric array=w398) -> (sum=w401:u8)
            n301 = Concatenate Strings("输出脉冲数为:", w395, "\r\n") -> (w392:string)
            n302 = invoke on="接收:" class="Str" method="Append String"("string"=w392) -> ()  [unwired: 3 in, 4 out]
            n303 = Compound Arithmetic op=ADD(w407, w401, w406, w406, w406, w406, w406, w406, w406, w406) -> (w410:u8)
            n304 = Type Cast(x=w396) -> (*(type *) &x=w399:string)  [unwired: 1 in]
            n305 = Type Cast(x=u8 170) -> (*(type *) &x=w409:string)  [unwired: 1 in]
            n306 = Type Cast(x=w407) -> (*(type *) &x=w408:string)  [unwired: 1 in]
            n307 = Type Cast(x=w406) -> (*(type *) &x=w404:string)  [unwired: 1 in]
            n308 = Type Cast(x=w410) -> (*(type *) &x=w403:string)  [unwired: 1 in]
            n309 = Concatenate Strings(w409, w408, w399, w404, w404, w404, w404, w404, w404, w404, w404, w403, "/") -> (w390:string)
            n310 = String Length(string=w390) -> (length=w389:i32)
            n311 = call "sio write.vi"("len"=w389, "buf"=w390, "port"=w391) -> ()  [unwired: 6 in, 3 out]
          }
        }
      }
    }
    n312 = case shown="真" "刷新按钮" {
      selector: "刷新按钮" -> [_ w63]
      frame False {
      }
      frame True {
        n313 = Not(x=w63) -> (.not. x?=w62:bool)
        n314 = property on="刷新按钮" class="Bool (严格)"("Value"=w62) -> ()  [unwired: 2 in, 2 out]
        n315 = call "SearchCom.vi"("使用注册表？"=w62) -> ("下拉列表项"=w64:cluster{"String":string, "Value":i32}[])  [unwired: 2 in]
        n316 = property on="串口号" class="Ring (严格)"("StringsAndValues[]"=w64) -> ()  [unwired: 2 in, 2 out]
      }
    }
  }
  n317 = stacked-sequence {
    frame #0 {
      n318 = Wait (ms)(milliseconds to wait=u32 20) -> ()  [unwired: 1 out]
    }
    frame #1 {
      # "调整启动时的前面板尺寸边界"
      # "应当等程序启动之后再执行这一步→_→"
      n319 = Call Chain ("调用链")() -> (call chain=w415:string[])
      n320 = Index Array(array=w415, index=0) -> (element=w413:string)
      n321 = Open VI Reference(vi path=w413) -> (vi reference=w425:refnum<vi>)  [unwired: 1 in, 5 out]
      n322 = property class="VI"(reference=w425) -> ("Front Panel.PanelBounds"=w422:T4)  [unwired: 1 in, 2 out]
      n323 = property class="VI"(reference=w425) -> (reference out=w426:refnum<vi>, "Minimum Panel Size"=w416:T5)  [unwired: 1 in, 1 out]
      n324 = Unbundle By Name(w416) -> ("Horizontal"=w423:i16, "Vertical"=w420:i16)
      n325 = Unbundle By Name(w422) -> ("Left"=w424:i16, "Top"=w419:i16)
      n326 = Add(x=w423, y=w424) -> (x+y=w421:i16)
      n327 = Add(x=w420, y=w419) -> (x+y=w418:i16)
      n328 = Bundle By Name(cluster=w422, "Right"=w421, "Bottom"=w418) -> (w417:T4)
      n329 = property class="VI"(reference=w426, "Front Panel.PanelBounds"=w417) -> (reference out=w427:refnum<vi>)  [unwired: 1 in, 1 out]
      n330 = Close Reference(reference=w427) -> ()  [unwired: 1 in, 1 out]
    }
    frame #2 {
      w430 = i16 0
      # "自动调整窗格原点"
      n331 = property on="Pane" class="Pane"() -> ("Origin"=w429:T5)  [unwired: 2 in, 2 out]
      n332 = Bundle By Name(cluster=w429, "Horizontal"=w430, "Vertical"=w430) -> (w428:T5)
      n333 = property on="Pane" class="Pane"("Origin"=w428) -> ()  [unwired: 2 in, 2 out]
    }
    frame #3 {
      n334 = property on="接收:" class="Str"("Value"="硬石电子http://www.ing10bbs.com/\n            携手合作,共创未来\n") -> ()  [unwired: 2 in, 2 out]
      n335 = call "SearchCom.vi"() -> ("下拉列表项"=w431:cluster{"String":string, "Value":i32}[])  [unwired: 3 in]
      n336 = property on="串口号" class="Ring (严格)"("StringsAndValues[]"=w431) -> ()  [unwired: 2 in, 2 out]
      n337 = property on="串口号" class="Ring (严格)"("DisabledEnum"=T2."Enabled" ("禁用")) -> ()  [unwired: 2 in, 2 out]
    }
  }
